vi "未命名 1.vi"() -> ()   [LabVIEW 2020]
uses:
  <vilib>/addons/database/Connection.llb/DB Tools Open Connec (String).vi
  <vilib>/addons/database/NI_Database_API.lvlib
panel:
  out "左正小结果":string
  out "正向空载最小扭矩(Nm)  2":dbl format="%.3g"
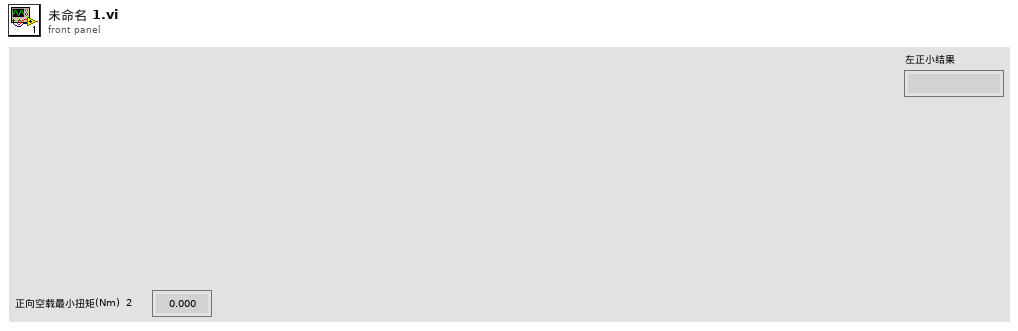
[diagram p1: front panel]
types:
  T1 = cluster{i64, i64, string, "正向空载最小扭矩(Nm)  2":dbl, "正向空载最小扭矩(Nm)  2":dbl, "正向空载最小扭矩(Nm)  2":dbl, string, "左正小结果 ":string}
  T2 = cluster{i64, i64, string, "正向空载最小扭矩(Nm)  2":dbl, "正向空载最小扭矩(Nm)  2":dbl, "正向空载最小扭矩(Nm)  2":dbl, string, "左正小结果 ":string}[]
  T3 = typedef "NI_Database_API.lvlib/Conn ObjectReference.ctl" = refnum<k1>
  T4 = cluster{i64, i64, "正向空载最小扭矩(Nm)  2":dbl, "正向空载最小扭矩(Nm)  2":dbl, "正向空载最小扭矩(Nm)  2":dbl, string, "左正小结果 ":string}
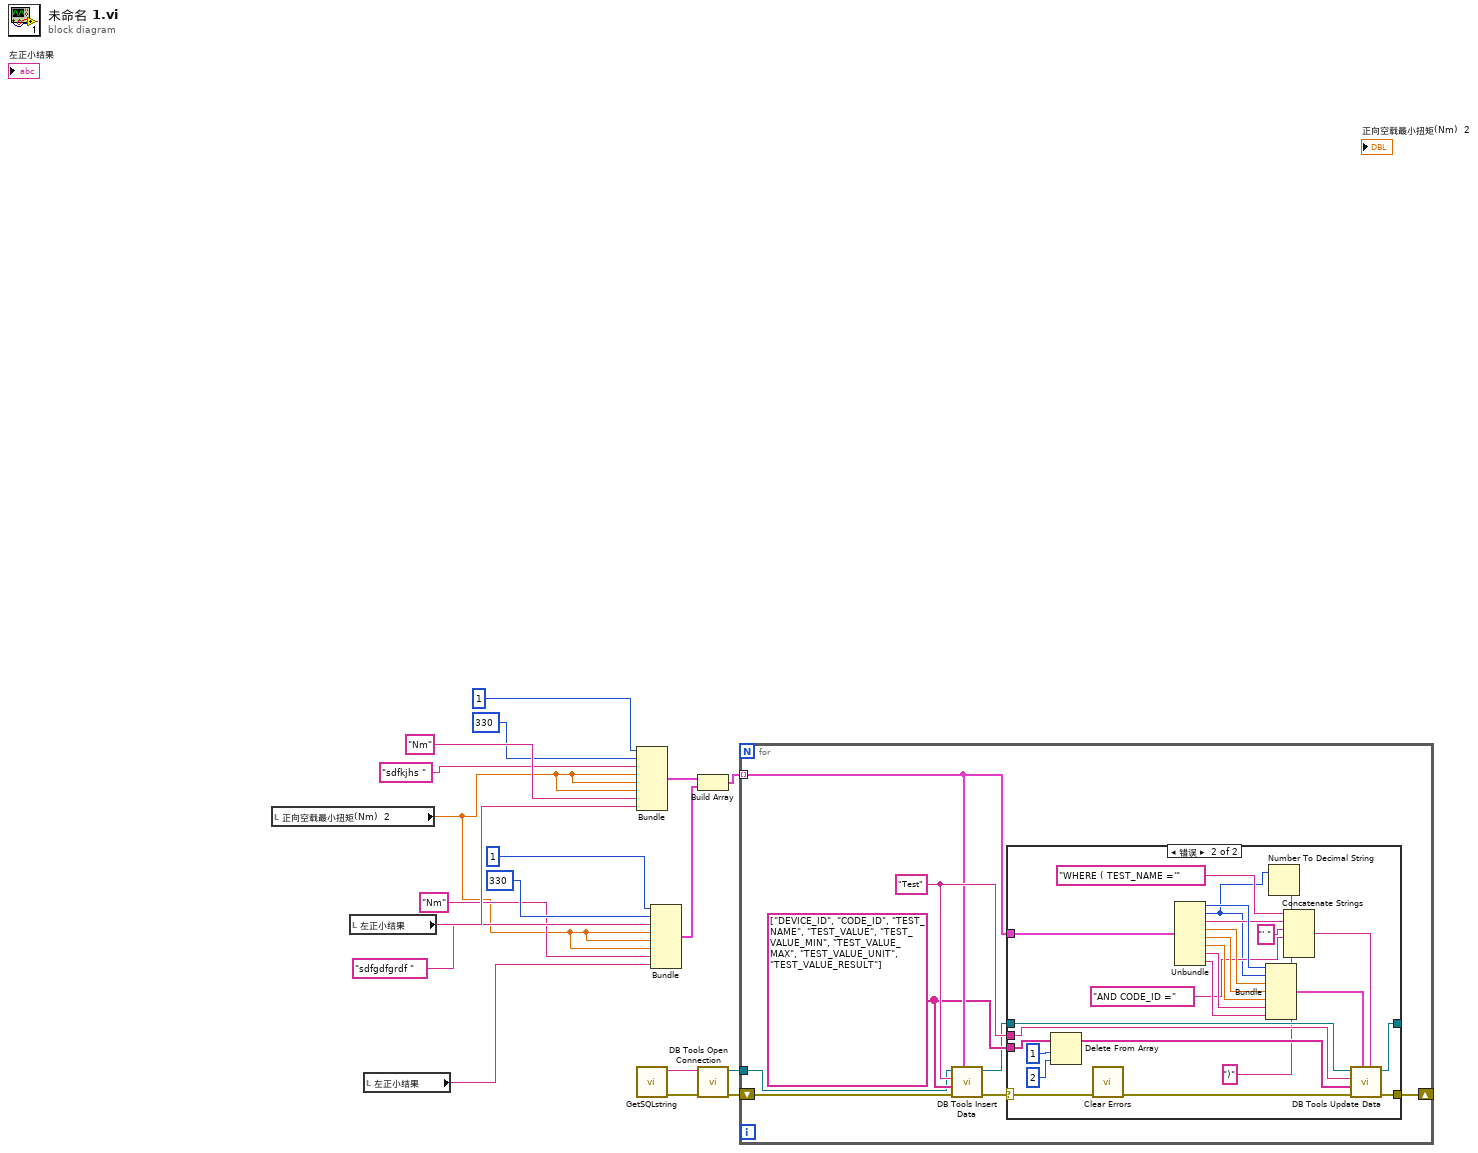
[diagram p0: block diagram]
diagram:
  n1 = local read "正向空载最小扭矩(Nm)  2"() -> (w2:dbl)
  n2 = local read "左正小结果"() -> (w12:string)
  n3 = local read "左正小结果"() -> (w4:string)
  n4 = Bundle(i64 1, i64 330, "sdfkjhs ", "正向空载最小扭矩(Nm)  2"=w2, "正向空载最小扭矩(Nm)  2"=w2, "正向空载最小扭矩(Nm)  2"=w2, "Nm", "左正小结果"=w12) -> (w11:T1)  [unwired: 1 in]
  n5 = call "GetSQLstring.vi"() -> ("错误输出"=w16:errorcluster, "连接字符串"=w17:string)  [unwired: 10 in]
  n6 = Bundle(i64 1, i64 330, "sdfgdfgrdf ", "正向空载最小扭矩(Nm)  2"=w2, "正向空载最小扭矩(Nm)  2"=w2, "正向空载最小扭矩(Nm)  2"=w2, "Nm", "左正小结果"=w4) -> (w1:T1)  [unwired: 1 in]
  n7 = Build Array(w11, w1) -> (w14:T2)
  n8 = call-poly <vilib>:"DB Tools Open Connection.vi"("error in (no error)"=w16, "connection information"=w17) -> ("error out"=w18:errorcluster, "connection reference"=w15:T3)  [unwired: 6 in]
  n9 = for {
    tunnel: w14 -> [w23] mode=indexing
    tunnel: w15 -> [w21]
    shift-right: [w19] -> _
    shift-left: w18 -> [w26]
    w22 = string[] ["DEVICE_ID", "CODE_ID", "TEST_NAME", "TEST_VALUE", "TEST_VALUE_MIN", "TEST_VALUE_MAX", "TEST_VALUE_UNIT", "TEST_VALUE_RESULT"] ("columns")
    w24 = "Test" ("table")
    n10 = call <vilib>:"DB Tools Insert Data.vi"("data"=w23, "error in (no error)"=w26, "columns"=w22, "table"=w24, "connection reference"=w21) -> ("error out"=w25:errorcluster, "connection reference out"=w20:T3)  [unwired: 5 in]
    n11 = case shown="错误" w25 {
      selector: w25 -> [w27 w53]
      tunnel: w22 -> [_ w50]
      tunnel: w20 -> [w28 w35]
      tunnel: w24 -> [_ w54]
      tunnel: w23 -> [_ w44]
      tunnel: [w28 w34] -> _
      tunnel: [w27 w33] -> w19
      frame No Error {
      }
      frame Error {
        n12 = Delete From Array(array=w50, length=1 ("长度"), index=2 ("索引")) -> (array with subset deleted=w51:string[])  [unwired: 1 out]
        n13 = call <vilib>:"Clear Errors.vi"("error in (no error)"=w53) -> ("error out"=w52:errorcluster)  [unwired: 5 in, 1 out]
        n14 = Unbundle(w44) -> (w43:i64, w31:i64, w36:string, "正向空载最小扭矩(Nm)  2"=w42:dbl, "正向空载最小扭矩(Nm)  2"=w41:dbl, "正向空载最小扭矩(Nm)  2"=w40:dbl, w39:string, "左正小结果"=w38:string)
        n15 = Bundle(w43, w31, "正向空载最小扭矩(Nm)  2"=w42, "正向空载最小扭矩(Nm)  2"=w41, "正向空载最小扭矩(Nm)  2"=w40, w39, "左正小结果"=w38) -> (w37:T4)  [unwired: 1 in]
        n16 = Number To Decimal String(number=w31) -> (decimal integer string=w30:string)  [unwired: 1 in]
        n17 = Concatenate Strings("WHERE ( TEST_NAME ='" ("condition"), w36, "' ", "AND CODE_ID =" ("condition"), w30, ")" ("condition")) -> (w46:string)
        n18 = call <vilib>:"DB Tools Update Data.vi"("condition"=w46, "data"=w37, "error in (no error)"=w52, "columns"=w51, "table"=w54, "connection reference"=w35) -> ("error out"=w33:errorcluster, "connection reference out"=w34:T3)  [unwired: 4 in]
      }
    }
  }
